vi "Anritsu VNA Determine Number of Ports.vi"(9 "Parameter":cluster{"Response Port":i8, "Stimulus Port":i8}) -> (1 "Number of Ports":i8)   [LabVIEW 2011]
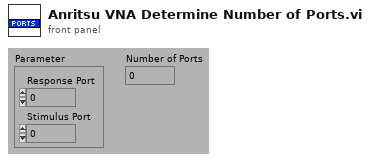
[diagram p1: front panel]
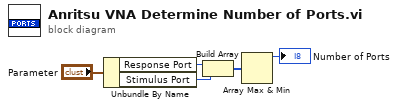
[diagram p0: block diagram]
diagram:
  n1 = Unbundle By Name("Parameter") -> ("Response Port"=w5:i8, "Stimulus Port"=w4:i8)
  n2 = Build Array(w5, w4) -> (w3:i8[])
  n3 = Array Max & Min(array=w3) -> (max value=→"Number of Ports":i8)  [unwired: 3 out]
